vi "Verify Credentials.vi"(4 "Access Token Secret (In)":string, 6 "Access Token (In)":string, 8 "error in (no error)":errorcluster, 10 "Consumer Secret":string, 11 "Consumer Key":string) -> (0 "error out":errorcluster, 1 "Screen Name":string, 2 "Success?":bool, 3 "HTTP Error Code":i32)   [LabVIEW 2011, in "i3-twitter.lvlib"]
doc: "Attempts to verify the supplied credentials with Twitter.com. If the credential are invalid, the user will be asked to enter his username and password.\n\nhttps://api.twitter.com/1/account/verify_credentials.xml"
uses:
  i3-twitter.lvlib
  i3-oauth/Controls/Signature Method.ctl
  i3-oauth/Controls/HTTP Method.ctl
  i3-json/JSON Parsing/Get Object Parameter Files/Get Object Parameter - String.vi
  <vilib>/httpClient/LabVIEWHTTPClient.lvlib
  i3-oauth/i3-oauth.lvlib
  i3-json/i3-json.lvlib
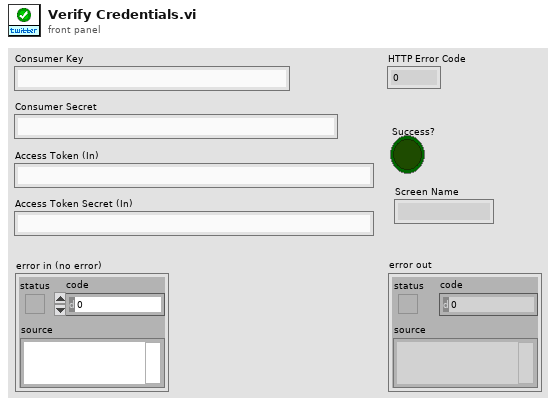
[diagram p1: front panel]
types:
  T1 = typedef "i3-oauth.lvlib/Signature Method.ctl" = enum16{"HMAC-MD5", "HMAC-SHA1", "HMAC-SHA224", "HMAC-SHA256", "HMAC-SHA384", "HMAC-SHA512"}
  T2 = typedef "i3-oauth.lvlib/HTTP Method.ctl" = enum16{"GET", "POST", "PUT", "DELETE"}
  T3 = typedef "i3-oauth.lvlib/OAuth Handle.ctl" = cluster{"Signature Method":T1, "Version":string, "Client":T4, "Access":T4}
  T4 = typedef "i3-oauth.lvlib/Credentials.ctl" = cluster{"Token":string, "Secret":string}
  T5 = typedef "LabVIEWHTTPClient.lvlib/ClientHandle.ctl" = refnum<k1>
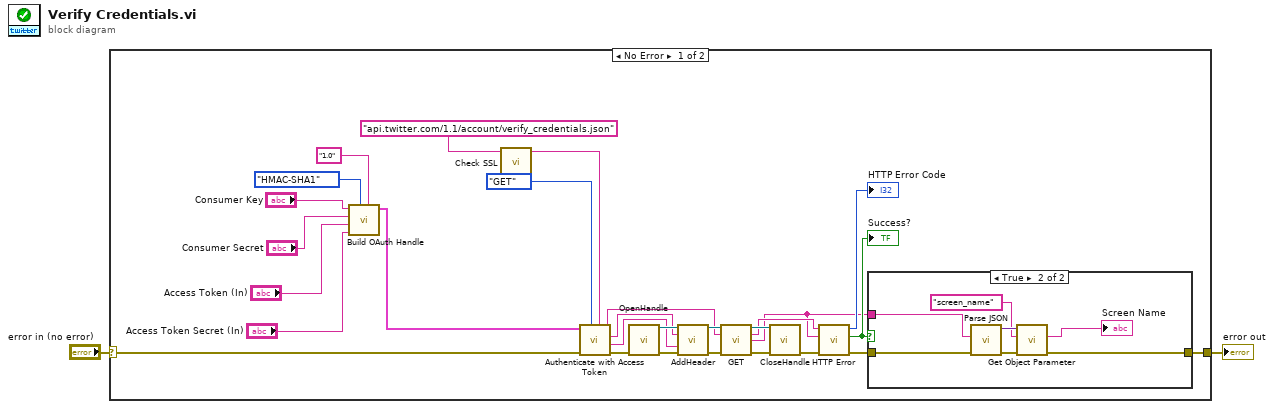
[diagram p0: block diagram]
diagram:
  n1 = case shown="No Error" "error in (no error)" {
    selector: "error in (no error)" -> [w14 w39]
    tunnel: [w19 w39] -> w2
    frame No Error {
      n2 = call "Build OAuth Handle.vi"("Version (1.0)"="1.0", "Signature Method (HMAC-SHA1)"=Signature_Method."HMAC-SHA1", "Access Secret"="Access Token Secret (In)", "Access Token"="Access Token (In)", "Client Secret"="Consumer Secret", "Client Token"="Consumer Key") -> ("OAuth Handle"=w3:T3)  [unwired: 5 in]
      n3 = call "Check SSL.vi"("Input URL"="api.twitter.com/1.1/account/verify_credentials.json" ("Base URL")) -> ("Output URL"=w10:string)  [unwired: 8 in]
      n4 = call "Authenticate with Access Token.vi"("Base URL"=w10, "HTTP Method"=HTTP_Method."GET", "error in (no error)"=w14, "OAuth Handle"=w3) -> ("error out"=w15:errorcluster, "Header Value"=w21:string, "Header Parameter"=w23:string, "Full URL"=w13:string)  [unwired: 3 in, 1 out]
      n5 = call <vilib>:"OpenHandle.vi"("error in (no error)"=w15) -> ("client handle out"=w24:T5, "error out"=w16:errorcluster)  [unwired: 13 in]
      n6 = call <vilib>:"AddHeader.vi"("client handle"=w24, "header"=w23, "value"=w21, "error in (no error)"=w16) -> ("client handle out"=w22:T5, "error out"=w25:errorcluster)  [unwired: 10 in]
      n7 = call <vilib>:"GET.vi"("client handle"=w22, "url"=w13, "error in (no error)"=w25) -> ("client handle out"=w29:T5, "headers"=w28:string, "body"=w17:string, "error out"=w30:errorcluster)  [unwired: 9 in]
      n8 = call <vilib>:"CloseHandle.vi"("client handle"=w29, "error in (no error)"=w30) -> ("error out"=w27:errorcluster)  [unwired: 13 in]
      n9 = call "HTTP Error.vi"("error in (no error)"=w27, "Body"=w17, "Header"=w28) -> ("error out"=w20:errorcluster, "Success?"=w18:bool, "HTTP Error Code"=→"HTTP Error Code":i32)  [unwired: 6 in]
      "Success?" <- w18
      n10 = case shown="True" w18 {
        tunnel: w17 -> [_ w38]
        tunnel: w20 -> [w31 w35]
        tunnel: [w31 w33] -> w19
        frame False {
        }
        frame True {
          n11 = call "Parse JSON.vi"("error in (no error)"=w35, "JSON String"=w38) -> ("error out"=w34:errorcluster, "JSON Tree"=w37:variant)  [unwired: 6 in, 2 out]
          n12 = call-poly "Get Object Parameter.vi"("error in (no error)"=w34, "Parameter Name"="screen_name", "JSON Tree In (JSON Object)"=w37) -> ("error out"=w33:errorcluster, "String Value"=→"Screen Name":string)  [unwired: 5 in, 2 out]
        }
      }
    }
    frame Error {
    }
  }
  "error out" <- w2
